vi "Save angle.vi"(2 "Angle graphs":string, 3 "Angle data":string, 4 "Elbow CircStat":dbl[](array[numeric]), 5 "Step":dbl, 6 "Shoulder CircStat Counterclockwise":dbl[](array[numeric]), 7 "Animal Number":dbl, 8 "Angle mean subtracted (output)":dbl[][](array[numeric]), 9 "Shoulder-Elbow angle data":dbl[][](array[numeric]), 10 "Pos, Neg increments":dbl[][](array[numeric]), 11 "Angle RMS":dbl[][](array[numeric])) -> ()   [LabVIEW 2020]
panel:
  out "concatenated string 3":string
  out "concatenated string 2":string
  out "Angle waveforms":dbl[][](array[numeric])
  out "Angle Data":dbl[][](array[numeric])
  out "Angle Data":dbl[][](array[numeric])
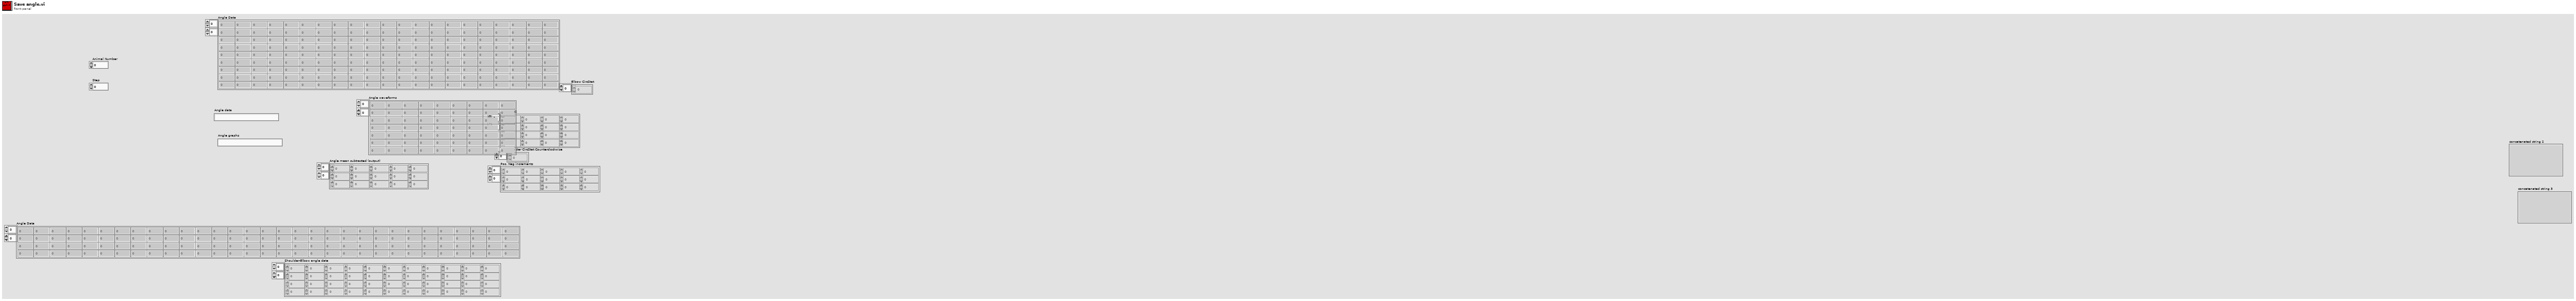
[diagram p1: front panel]
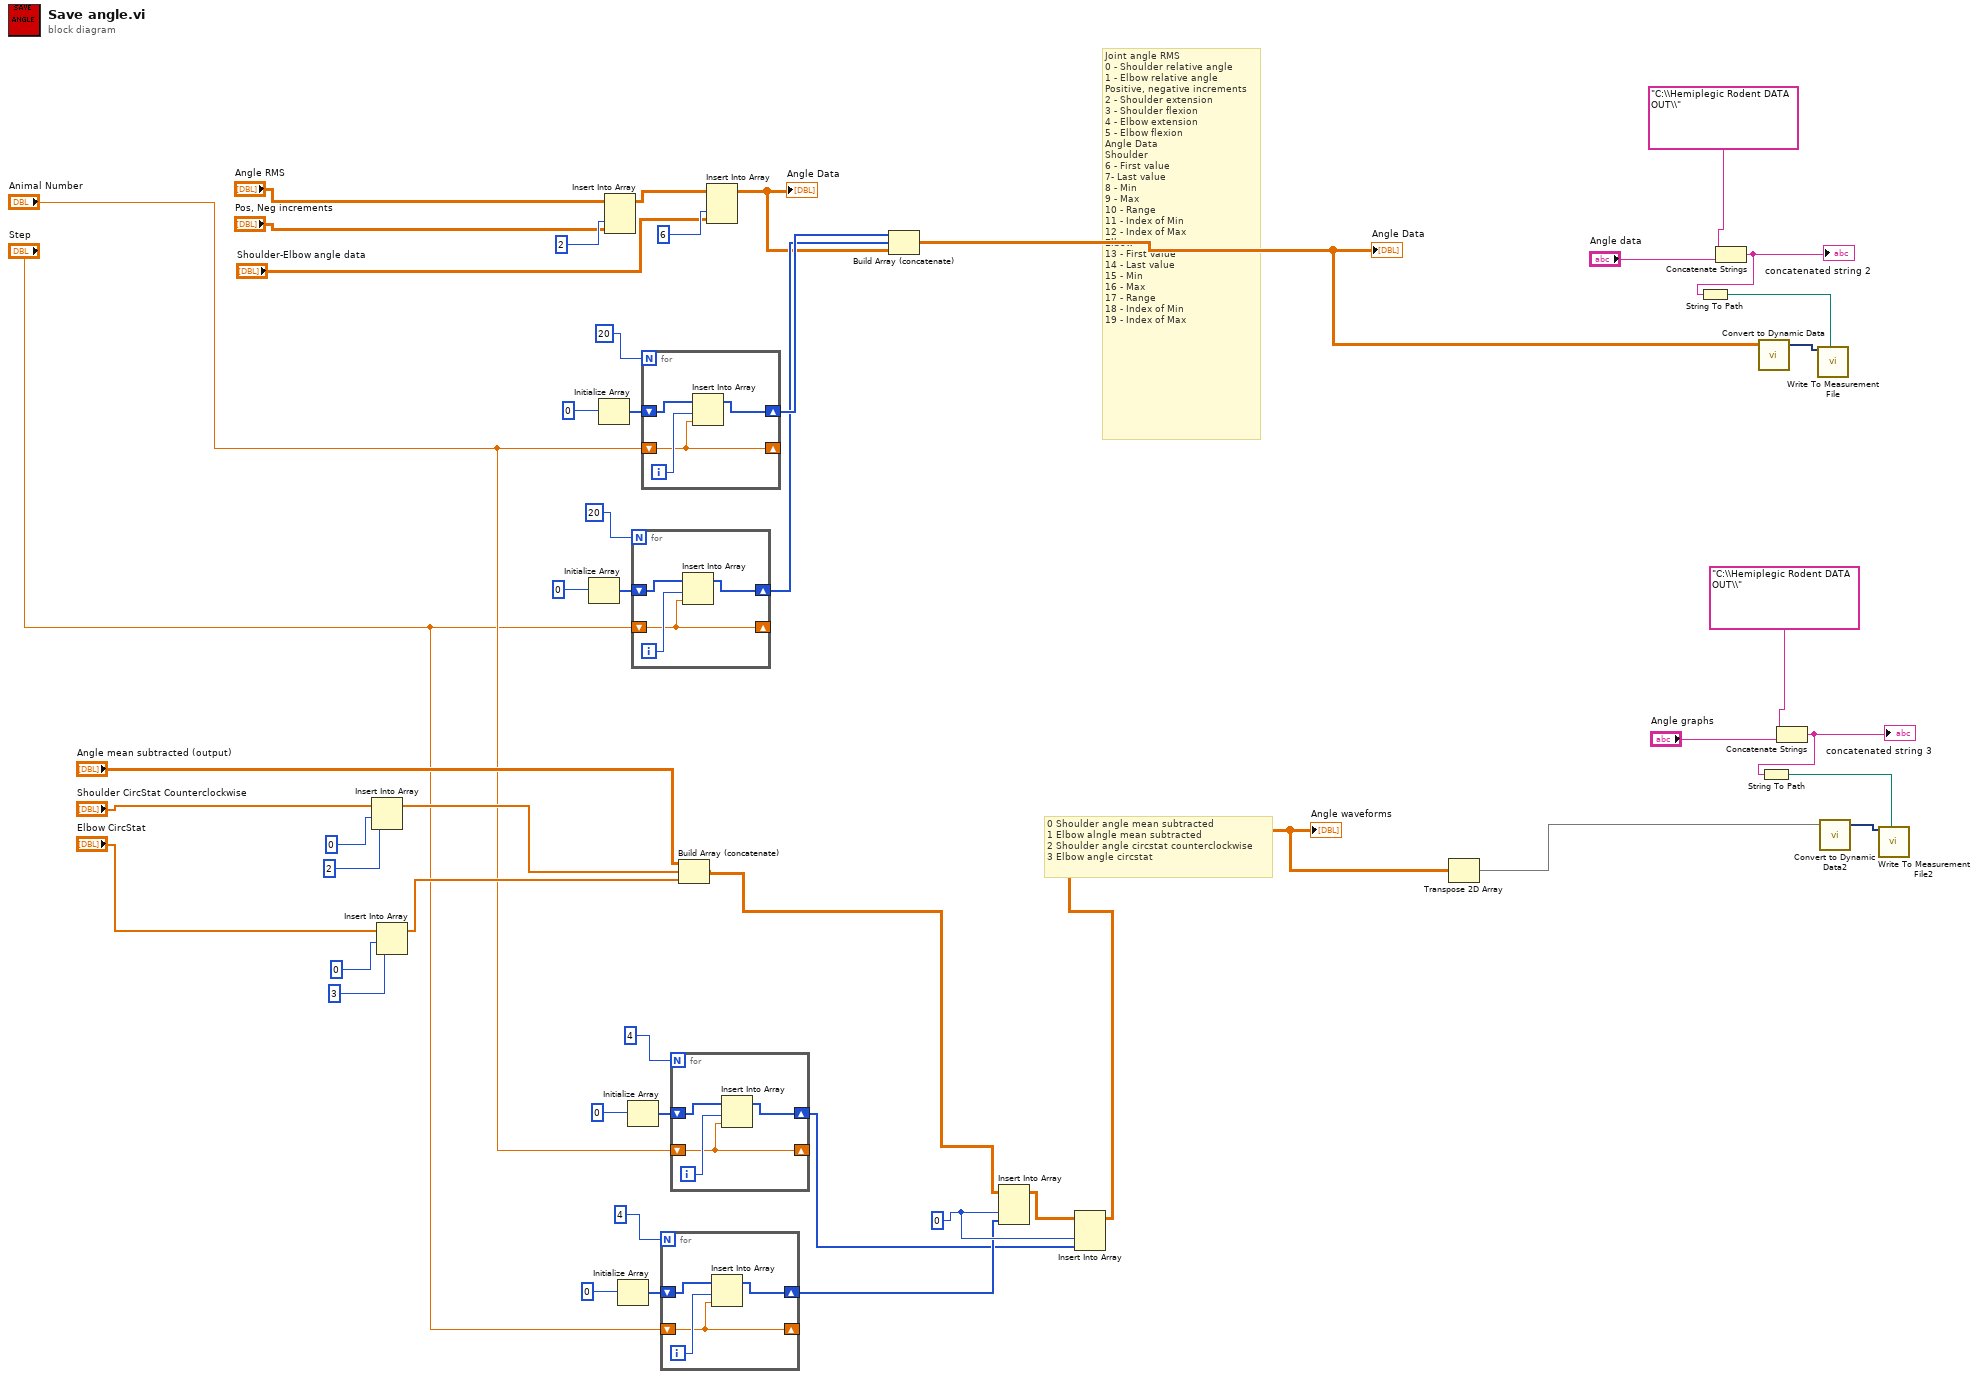
[diagram p0: block diagram]
diagram:
  w18 = 0
  # "0 Shoulder angle mean subtracted\n1 Elbow alngle mean subtracted\n2 Shoulder angle circstat counterclockwise\n3 Elbow angle circstat"
  # "Joint angle RMS\n0 - Shoulder relative angle\n1 - Elbow relative angle\nPositive, negative increments\n2 - Shoulder extension\n3 - Shoulder flexion\n4 - Elbow extension\n5 - Elbow flexion\nAngle Data\nShoulder\n6 - First value\n7- Last value\n8 - Min\n9 - Max\n10 - Range\n11 - Index of Min\n12 - Index of Max\nElbow\n13 - First value\n14 - Last value\n15 - Min\n16 - Max\n17 - Range\n18 - Index of Min\n19 - Index of Max"
  n1 = Insert Into Array(array="Shoulder CircStat Counterclockwise", index=0, new element=2) -> (w29:dbl[])
  n2 = Insert Into Array(array="Elbow CircStat", index=0, new element=3) -> (w28:dbl[])
  n3 = Initialize Array(0) -> (w40:i32[])  [unwired: 1 in]
  n4 = Initialize Array(0) -> (w43:i32[])  [unwired: 1 in]
  n5 = Insert Into Array(array="Angle RMS", index (col)=2, new element="Pos, Neg increments") -> (w46:dbl[][])  [unwired: 1 in]
  n6 = Initialize Array(0) -> (w22:i32[])  [unwired: 1 in]
  n7 = Initialize Array(0) -> (w25:i32[])  [unwired: 1 in]
  n8 = for {
    N: 20 -> [_]
    shift-right: [w52] -> w38
    shift-left: w40 -> [w53]
    shift-right: [w51] -> _
    shift-left: "Step" -> [w51]
    i -> [w54]
    n9 = Insert Into Array(array=w53, index=w54, new element=w51) -> (w52:i32[])
  }
  n10 = for {
    N: 20 -> [_]
    shift-right: [w56] -> w39
    shift-left: w43 -> [w57]
    shift-right: [w55] -> _
    shift-left: "Animal Number" -> [w55]
    i -> [w58]
    n11 = Insert Into Array(array=w57, index=w58, new element=w55) -> (w56:i32[])
  }
  n12 = for {
    N: 4 -> [_]
    shift-right: [w60] -> w16
    shift-left: w22 -> [w61]
    shift-right: [w59] -> _
    shift-left: "Step" -> [w59]
    i -> [w62]
    n13 = Insert Into Array(array=w61, index=w62, new element=w59) -> (w60:i32[])
  }
  n14 = for {
    N: 4 -> [_]
    shift-right: [w64] -> w15
    shift-left: w25 -> [w65]
    shift-right: [w63] -> _
    shift-left: "Animal Number" -> [w63]
    i -> [w66]
    n15 = Insert Into Array(array=w65, index=w66, new element=w63) -> (w64:i32[])
  }
  n16 = Build Array (concatenate)("Angle mean subtracted (output)", w29, w28) -> (w17:dbl[][])
  n17 = Insert Into Array(array=w46, index (col)=6, new element="Shoulder-Elbow angle data") -> (w37:dbl[][])  [unwired: 1 in]
  "Angle Data" <- w37
  n18 = Build Array (concatenate)(w39, w38, w37) -> (w8:dbl[][])
  "Angle Data" <- w8
  n19 = Insert Into Array(array=w17, index (col)=w18, new element=w16) -> (w19:dbl[][])  [unwired: 1 in]
  n20 = Insert Into Array(array=w19, index (col)=w18, new element=w15) -> (w2:dbl[][])  [unwired: 1 in]
  "Angle waveforms" <- w2
  n21 = Transpose 2D Array(2D array=w2) -> (transposed array=w1:dbl[][])
  n22 = Concatenate Strings("C:\\Hemiplegic Rodent DATA OUT\\" ("name"), "Angle data") -> (w12:string)
  "concatenated string 2" <- w12
  n23 = String To Path(string=w12) -> (path=w10:path)
  n24 = call "Convert to Dynamic Data"("2D Array"=w8) -> ("Dynamic Data Type"=w9:dynamicdata)  [unwired: 3 in]
  n25 = Concatenate Strings("C:\\Hemiplegic Rodent DATA OUT\\" ("name"), "Angle graphs") -> (w6:string)
  "concatenated string 3" <- w6
  n26 = String To Path(string=w6) -> (path=w4:path)
  n27 = call "Write To Measurement File"("Signals"=w9, "Filename"=w10) -> ()  [unwired: 15 in, 3 out]
  n28 = call "Convert to Dynamic Data2"("2D Array"=w1) -> ("Dynamic Data Type"=w3:dynamicdata)  [unwired: 3 in]
  n29 = call "Write To Measurement File2"("Signals"=w3, "Filename"=w4) -> ()  [unwired: 15 in, 3 out]
